vi "GT Get Watch Info.vi"(8 "error in (no error)":errorcluster caption="错误输入（无错误）", 10 "pInfo":T1, 11 "cardNum":i16) -> (0 "error out":errorcluster caption="错误输出", 2 "pInfo out":T1, 3 "function return":i16)   [LabVIEW 2020, in "gts1.lvlib"]
doc: "GT_API GT_GetWatchInfo(short cardNum,TWatchInfo *pInfo);"
uses:
  gts1.lvlib
  dll/32bit/multi_card/gts.dll
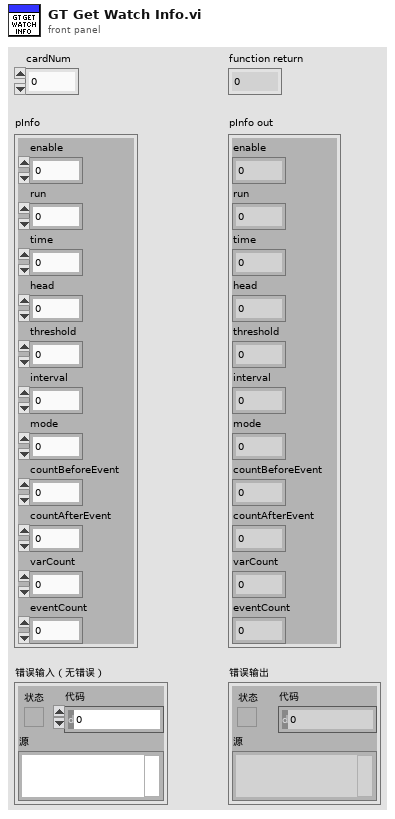
[diagram p1: front panel]
types:
  T1 = cluster{"enable":i16, "run":i16, "time":u32, "head":u32, "threshold":u32, "interval":i16, "mode":i16, "countBeforeEvent":u16, "countAfterEvent":u16, "varCount":u16, "eventCount":u16}
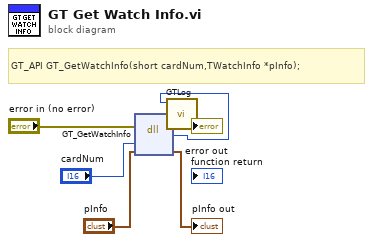
[diagram p0: block diagram]
diagram:
  # "GT_API GT_GetWatchInfo(short cardNum,TWatchInfo *pInfo);"
  n1 = dll-call lib="C:/1228/dll/32bit/multi_card/gts.dll" fn="GT_GetWatchInfo"(error in="error in (no error)", "cardNum"="cardNum", "pInfo"="pInfo") -> (error out=w3:errorcluster, w1:i16, "pInfo"=→"pInfo out":T1)  [unwired: 3 in, 1 out]
  n2 = call "GTLog.vi"("error in (no error)"=w3, "Numeric"=w1) -> ("error out"=→"error out":errorcluster)  [unwired: 9 in]
